vi "Global.vi"() -> ()   [LabVIEW 2018]
panel:
  out "semaphore":T1
  in  "Bomb Control":bool
  in  "Emergency Stop":bool
  in  "Shutdown":bool
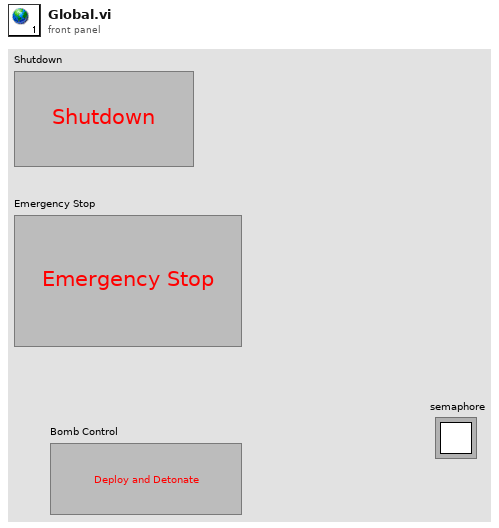
[diagram p1: front panel]
types:
  T1 = typedef "Semaphore RefNum" = refnum<k1>
diagram:
